vi "Load Slide Images from Disk.vi"(8 "error in (no error)":errorcluster) -> (0 "error out":errorcluster, 3 "Slides":picture[](array[picture]))   [LabVIEW 2020]
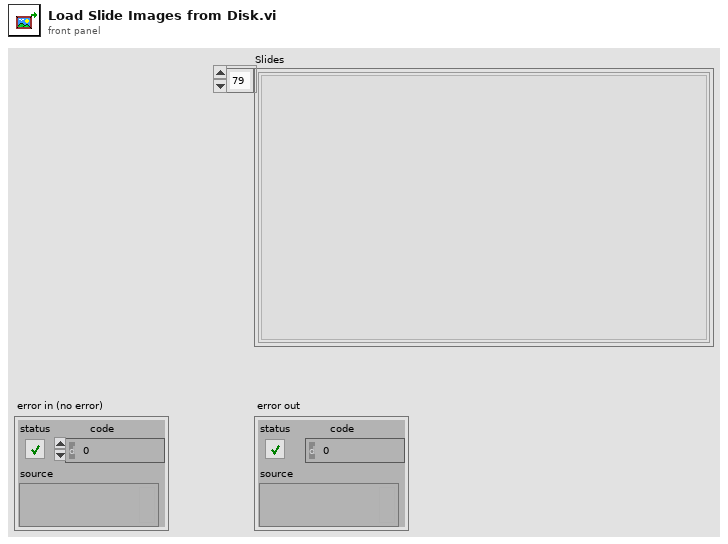
[diagram p1: front panel]
types:
  T1 = typedef "imagedata.ctl" = cluster{"image type":i32, "image depth":i32, "image":u8[], "mask":u8[], "colors":u32[], "Rectangle":cluster{"left":i16, "top":i16, "right":i16, "bottom":i16}}
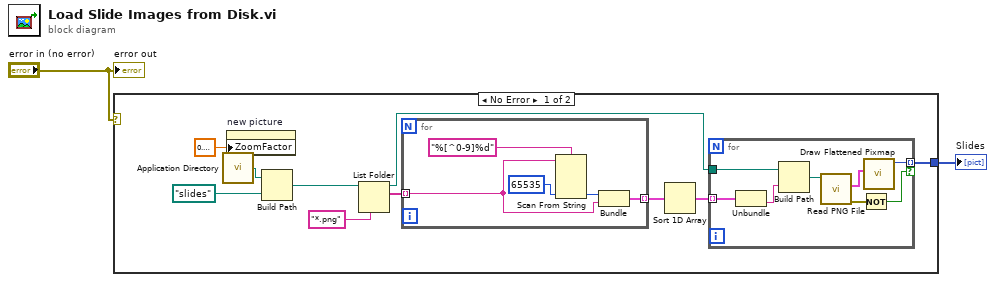
[diagram p0: block diagram]
diagram:
  n1 = case shown="No Error" "error in (no error)" {
    tunnel: [w9 _] -> w1
    frame No Error {
      n2 = call <vilib>:"Application Directory.vi"() -> ("Application Directory"=w10:path)
      n3 = property on="new picture" class="Pict"("ZoomFactor"=sgl 0.3 ("Zoom Factor")) -> ()  [unwired: 2 in, 2 out]
      n4 = Build Path(base path=w10, name or relative path=path "slides") -> (appended path=w11:path)
      n5 = List Folder(path=w11, pattern="*.png") -> (path out=w8:path, filenames=w6:string[])  [unwired: 2 in, 2 out]
      n6 = for {
        tunnel: w6 -> [w17] mode=indexing
        tunnel: [w15] -> w5 mode=indexing
        n7 = Scan From String(format string="%[^0-9]%d", input string=w17, default 2=u16 65535 ("default value 14")) -> (output 2=w13:u16)  [unwired: 4 in, 3 out]
        n8 = Bundle("default value 14"=w13, w17) -> (w15:cluster{"default value 14":u16, string})  [unwired: 1 in]
      }
      n9 = Sort 1D Array(array=w5) -> (sorted array=w4:cluster{"default value 14":u16, string}[])
      n10 = for {
        tunnel: w8 -> [w25]
        tunnel: [w22] -> w9 mode=indexing if=w21
        tunnel: w4 -> [w20] mode=indexing
        n11 = Unbundle(w20) -> (w18:string)  [unwired: 1 out]
        n12 = Build Path(base path=w25, name or relative path=w18) -> (appended path=w24:path)
        n13 = call <vilib>:"Read PNG File.vi"("path to PNG file"=w24) -> ("error out"=w19:errorcluster, "image data"=w23:T1)  [unwired: 8 in, 1 out]
        n14 = Not(x=w19) -> (.not. x?=w21:bool)
        n15 = call <vilib>:"Draw Flattened Pixmap.vi"("image data"=w23) -> ("new picture"=w22:picture)  [unwired: 8 in]
      }
    }
    frame Error {
    }
  }
  "Slides" <- w1
  "error out" <- "error in (no error)"
